vi "transconductance peak finder.vi"() -> ()   [LabVIEW 2016]
uses:
  <vilib>/Analysis/NI_AAL_SigProc.lvlib
  <vilib>/Analysis/NI_AALPro.lvlib
panel:
  out "Array":dbl[](array[numeric])=[7.098758556104314, -7.417307355510934]
  out "Locations":dbl[](array[numeric])=[51.13123598228449, 120.38395095984171]
  in  "width":i32=50 min=3
  in  "threshold":dbl=2.9996 format="%0.2f"
  out "size(s)":i32=173
  in  "reverse flattening array?":bool=TRUE
  out "Array 3":dbl[](array[numeric])=[-18.0004, -17.9998, -17.8137, -17.6036, -17.394, -17.1842, -16.9746, -16.7645, -16.5563, -16.3467, -16.1368, -15.9287, -15.7185, -15.5089, -15.2992, -15.0895, -14.8796, -14.67, -14.4602, -14.2521, -14.0423, -13.8327, -13.6229, -13.4133, -13.2049, -12.9953, -12.7852, -12.5773, -12.3674, -12.1577, -11.9476, -11.7381, -11.5296, -11.3198, -11.11, -10.9003, -10.6906, -10.4811, -10.2715, -10.062, -9.8526, -9.6425, -9.4322, -9.2222, -9.0141, -8.8044, -8.5948, -8.3845, -8.1753, -7.9654, -7.7557, -7.546, -7.3371, -7.1273, -6.9162, -6.7067, -6.4971, -6.2873, -6.0778, -5.8686, -5.6592, -5.4498, -5.2386, -5.0305, -4.8198, -4.6107, -4.4025, -4.1931, -3.9835, -3.7744, -3.5651, -3.3555, -3.1443, -2.9325, -2.7262, -2.5165, -2.3062, -2.0979, -1.8884, -1.6786, -1.468, -1.2578, -1.0491, -0.8365, -0.6289, -0.4182, -0.2096, 0.0006, 0.2111, 0.4199, 0.6277, 0.8368, 1.0468, 1.2564, 1.4643, 1.6748, 1.8832, 2.0939, 2.3032, 2.5144, 2.7237, 2.9332, 3.1425, 3.3523, 3.5631, 3.7729, 3.9819, 4.1914, 4.4021, 4.6101, 4.8206, 5.0302, 5.2398, 5.4493, 5.6584, 5.8691, 6.0784, 6.2876, 6.4968, 6.7057, 6.9171, 7.1262, 7.336, 7.5435, 7.7545, 7.9638, 8.1734, 8.3829, 8.5923, 8.802, 9.0116, 9.2206, 9.4321, 9.6403, 9.8516, 10.0609, 10.2704, 10.4793, 10.6894, 10.8992, 11.1084, 11.3181, 11.5275, 11.7369, 11.9465, 12.1554, 12.366, 12.5761, 12.7847, 12.995, 13.2052, 13.4153, 13.6251, 13.8337, 14.0433, 14.2535, 14.4621, 14.6726, 14.8827, 15.0929, 15.3032, 15.5113, 15.7213, 15.9304, 16.1402, 16.349, 16.559, 16.7671, 16.9778, 17.1861, 17.3978, 17.6064, 17.8158]
  in  "Array 2":dbl[](array[numeric])
  in  "length":i32=200
  in  "index":i32
  out "first peak":cluster{dbl[], "Best Linear Fit":dbl[]}[](graph)
  in  "threshold 2":dbl=60.0 format="%0.2f"
  in  "width 2":i32=42 min=3
  in  "B field array":dbl[](array[numeric])=[-18.0004, -17.9998, -17.8137, -17.6036, -17.394, -17.1842, -16.9746, -16.7645, -16.5563, -16.3467, -16.1368, -15.9287, -15.7185, -15.5089, -15.2992, -15.0895, -14.8796, -14.67, -14.4602, -14.2521, -14.0423, -13.8327, -13.6229, -13.4133, -13.2049, -12.9953, -12.7852, -12.5773, -12.3674, -12.1577, -11.9476, -11.7381, -11.5296, -11.3198, -11.11, -10.9003, -10.6906, -10.4811, -10.2715, -10.062, -9.8526, -9.6425, -9.4322, -9.2222, -9.0141, -8.8044, -8.5948, -8.3845, -8.1753, -7.9654, -7.7557, -7.546, -7.3371, -7.1273, -6.9162, -6.7067, -6.4971, -6.2873, -6.0778, -5.8686, -5.6592, -5.4498, -5.2386, -5.0305, -4.8198, -4.6107, -4.4025, -4.1931, -3.9835, -3.7744, -3.5651, -3.3555, -3.1443, -2.9325, -2.7262, -2.5165, -2.3062, -2.0979, -1.8884, -1.6786, -1.468, -1.2578, -1.0491, -0.8365, -0.6289, -0.4182, -0.2096, 0.0006, 0.2111, 0.4199, 0.6277, 0.8368, 1.0468, 1.2564, 1.4643, 1.6748, 1.8832, 2.0939, 2.3032, 2.5144, 2.7237, 2.9332, 3.1425, 3.3523, 3.5631, 3.7729, 3.9819, 4.1914, 4.4021, 4.6101, 4.8206, 5.0302, 5.2398, 5.4493, 5.6584, 5.8691, 6.0784, 6.2876, 6.4968, 6.7057, 6.9171, 7.1262, 7.336, 7.5435, 7.7545, 7.9638, 8.1734, 8.3829, 8.5923, 8.802, 9.0116, 9.2206, 9.4321, 9.6403, 9.8516, 10.0609, 10.2704, 10.4793, 10.6894, 10.8992, 11.1084, 11.3181, 11.5275, 11.7369, 11.9465, 12.1554, 12.366, 12.5761, 12.7847, 12.995, 13.2052, 13.4153, 13.6251, 13.8337, 14.0433, 14.2535, 14.4621, 14.6726, 14.8827, 15.0929, 15.3032, 15.5113, 15.7213, 15.9304, 16.1402, 16.349, 16.559, 16.7671, 16.9778, 17.1861, 17.3978, 17.6064, 17.8158]
  in  "Transconductance":T1(graph)
  in  "Transcond Intensity":dbl[][](graph)
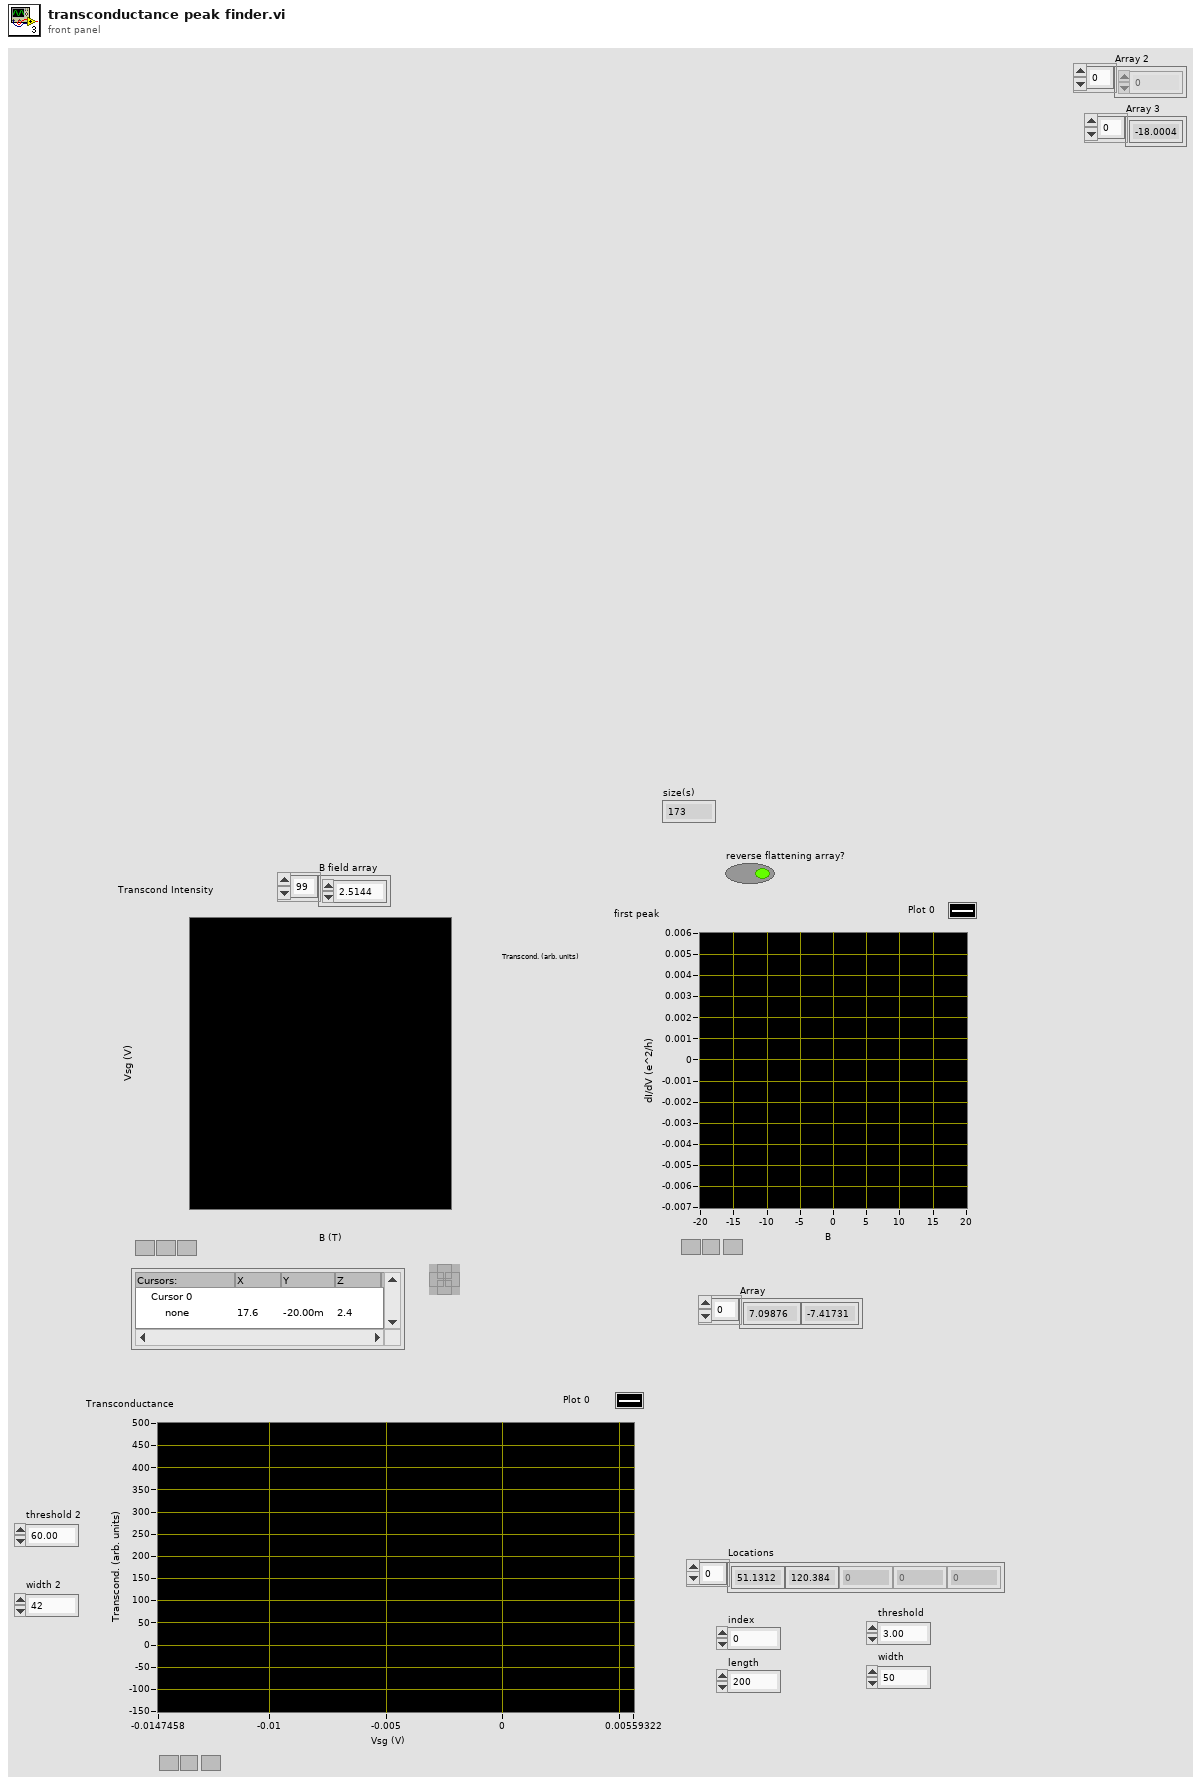
[diagram p1: front panel]
types:
  T1 = cluster{"Vfast":dbl[], "Decimated Array":dbl[]}[]
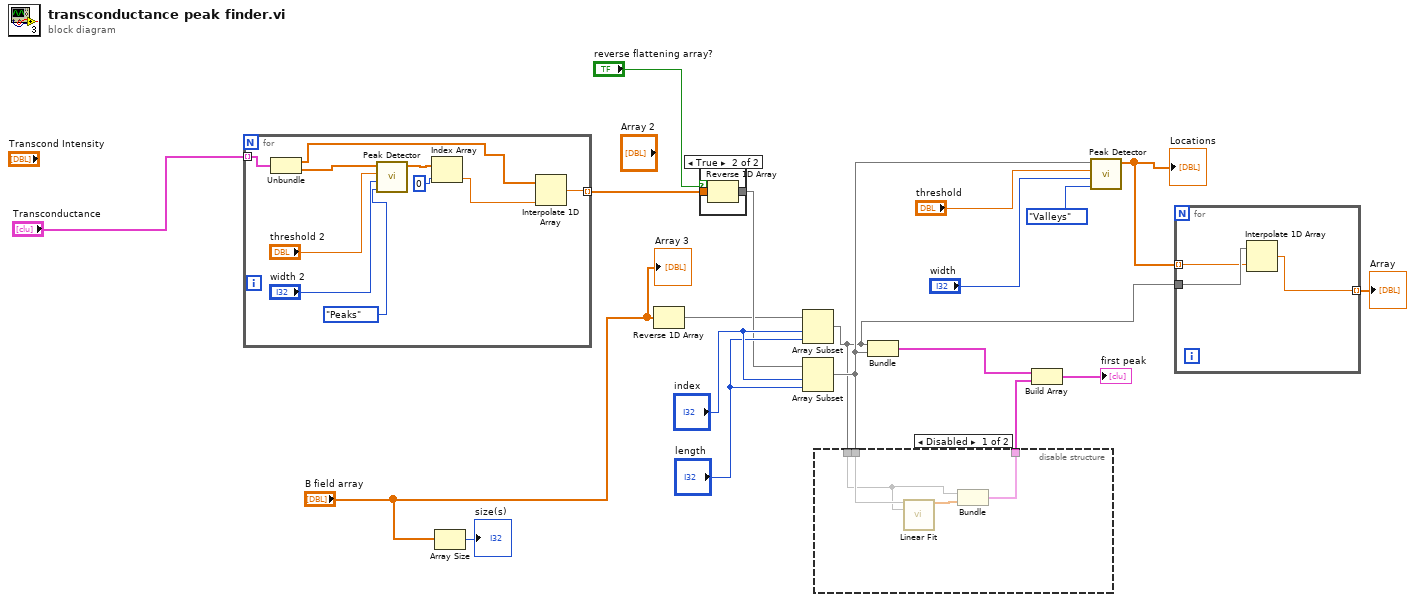
[diagram p0: block diagram]
diagram:
  n1 = for {
    tunnel: "Transconductance" -> [w29] mode=indexing
    tunnel: [w22] -> w11 mode=indexing
    n2 = Unbundle(w29) -> ("Vfast"=w24:dbl[], "Decimated Array"=w20:dbl[])
    n3 = call <vilib>:"Peak Detector.vi"("peaks/valleys"=enum32{"Peaks", "Valleys"}."Peaks", "width"="width 2", "threshold"="threshold 2", "X"=w20) -> ("Locations"=w28:dbl[])  [unwired: 3 in, 4 out]
    n4 = Index Array(array=w28, index=0) -> (element=w23:dbl)
    n5 = Interpolate 1D Array(1:w23, 2:w24) -> (0:w22:dbl)
  }
  n6 = Array Size(array="B field array") -> (size(s)=→"size(s)":i32)
  n7 = Reverse 1D Array(array="B field array") -> (reversed array=w13:dbl[])
  n8 = case shown="True" "reverse flattening array?" {
    tunnel: w11 -> [w30 w32]
    tunnel: [w30 w31] -> w14
    frame False {
    }
    frame True {
      n9 = Reverse 1D Array(array=w32) -> (reversed array=w31:dbl[])
    }
  }
  n10 = Array Subset(array=w13, index="index", length="length") -> (w3:dbl[])
  n11 = Array Subset(array=w14, index="index", length="length") -> (w6:dbl[])
  n12 = disable-structure shown="Disabled" {
    disable-tunnel: [w36 _] -> w15
    disable-tunnel: w6 -> [w34 _]
    disable-tunnel: w3 -> [w33 _]
    frame Disabled {
      n13 = call <vilib>:"Linear Fit.vi"("Y"=w34, "X"=w33) -> ("Best Linear Fit"=w35:dbl[])  [unwired: 9 in, 4 out]
      n14 = Bundle(w33, "Best Linear Fit"=w35) -> (w36:cluster{dbl[], "Best Linear Fit":dbl[]})  [unwired: 1 in]
    }
    frame Enabled {
    }
  }
  n15 = Bundle(w3, w6) -> (w17:cluster{dbl[], dbl[]})  [unwired: 1 in]
  n16 = Build Array(w17, w15) -> (→"first peak":cluster{dbl[], "Best Linear Fit":dbl[]}[])
  n17 = call <vilib>:"Peak Detector.vi"("peaks/valleys"=enum32{"Peaks", "Valleys"}."Valleys", "width"="width", "threshold"="threshold", "X"=w6) -> ("Locations"=w2:dbl[])  [unwired: 3 in, 4 out]
  "Locations" <- w2
  n18 = for {
    tunnel: w3 -> [w39]
    tunnel: w2 -> [w38] mode=indexing
    tunnel: [w37] -> w1 mode=indexing
    n19 = Interpolate 1D Array(1:w38, 2:w39) -> (0:w37:dbl)
  }
  "Array" <- w1
  "Array 3" <- "B field array"
